vi "_script_import_api_doc.vi"(10 "pattern":string="VI Description(CN) - *", 11 "md path":path) -> ()   [LabVIEW 2017]
uses:
  Communicable State Machine.lvlib
  _csmDoc/csmdoc.lvlib
panel:
  out "States":string
  out "appended array":path[](array[path])
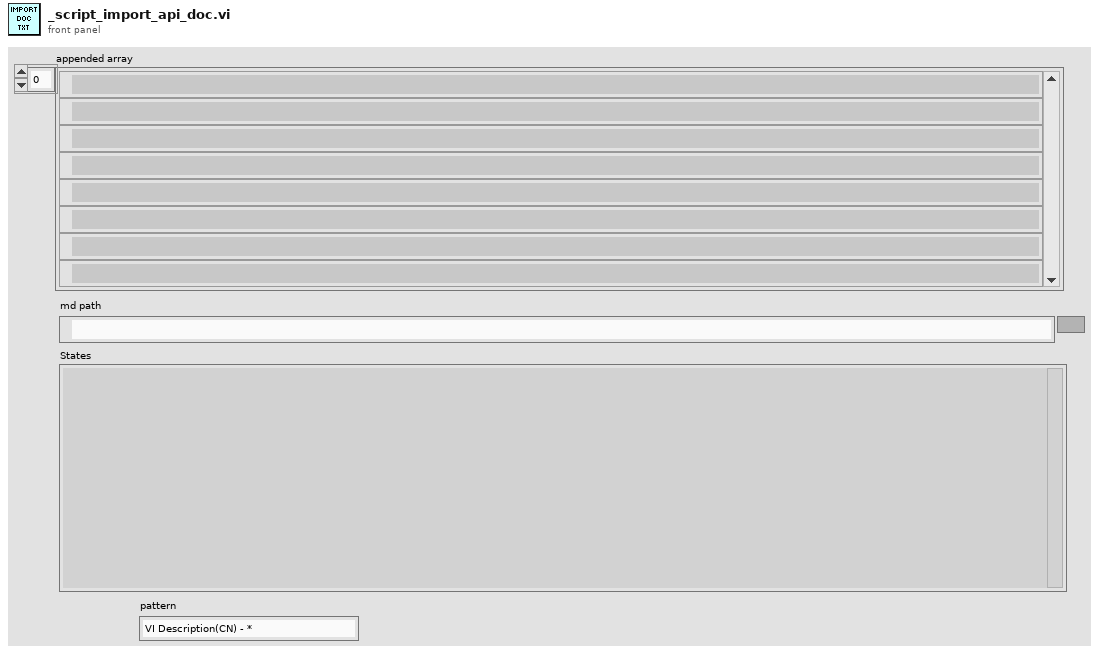
[diagram p1: front panel]
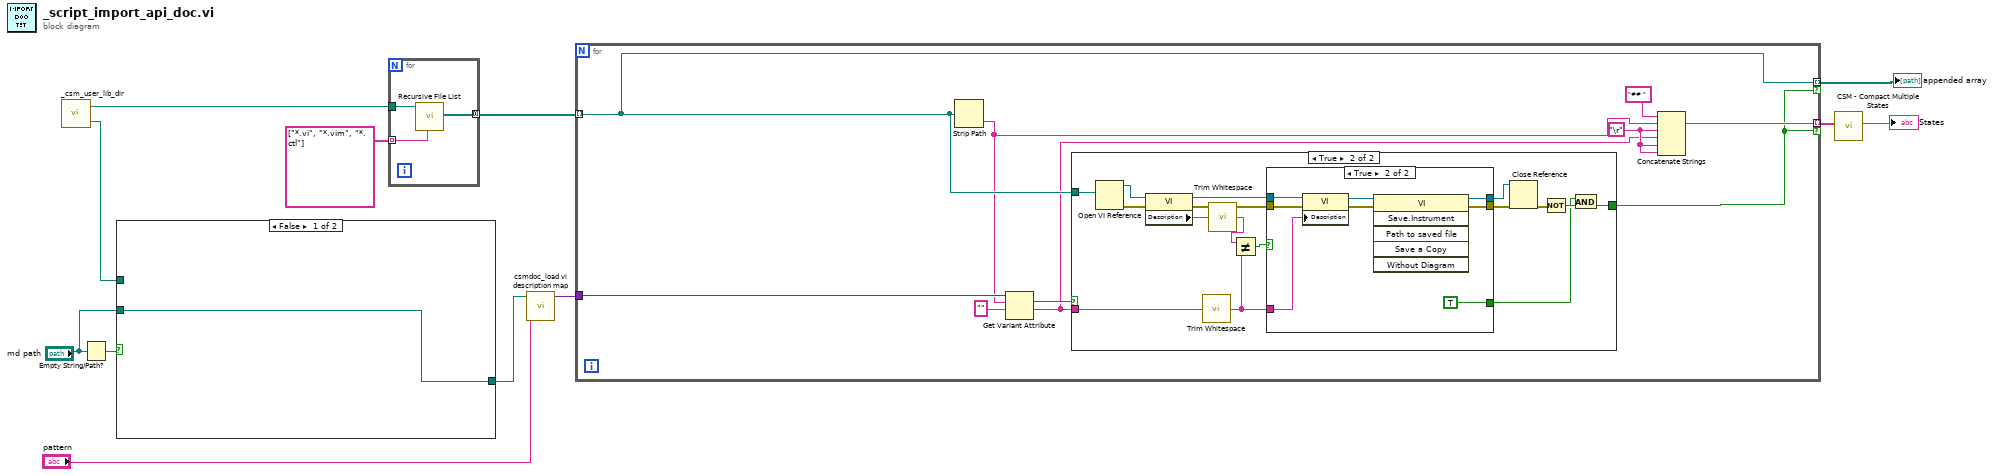
[diagram p0: block diagram]
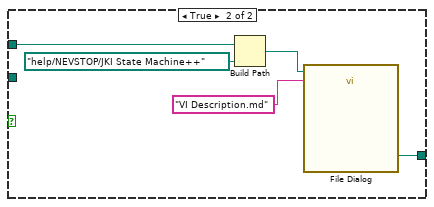
[diagram p2: hidden frame]
diagram:
  n1 = call "_csm_user_lib_dir.vi"() -> ("<LabVIEW>"=w4:path, "csm_user.lib_dir"=w5:path)  [unwired: 2 in]
  n2 = Empty String/Path?(string/path="md path") -> (empty?=w3:bool)
  n3 = case shown="False" w3 {
    tunnel: [w13 w16] -> w8
    tunnel: w4 -> [_ w14]
    tunnel: "md path" -> [w13 _]
    frame False {
    }
    frame True {
      n4 = Build Path(base path=w14, name or relative path=path "help/NEVSTOP/JKI State Machine++" ("Path")) -> (appended path=w17:path)
      n5 = call "File Dialog"("start path"=w17, "default name"="VI Description.md") -> ("selected path"=w16:path)  [unwired: 10 in, 3 out]
    }
  }
  n6 = for {
    tunnel: w5 -> [w21]
    tunnel: string[] ["*.vi", "*.vim", "*.ctl"] -> [w20] mode=indexing
    tunnel: [w19] -> w11 mode=concatenating
    n7 = call <vilib>:"Recursive File List.vi"("pattern"=w20, "Folder Path"=w21) -> ("All Files in Dir"=w19:path[])  [unwired: 5 in, 4 out]
  }
  n8 = call "csmdoc_load vi description map.vi"("pattern"="pattern", "Path"=w8) -> ("variant"=w9:variant)  [unwired: 7 in, 2 out]
  n9 = for {
    tunnel: w11 -> [w29] mode=indexing
    tunnel: [w31] -> w10 mode=indexing if=w30
    tunnel: w9 -> [w28]
    tunnel: [w29] -> w6 mode=indexing if=w30
    w26 = "\r"
    n10 = Strip Path(path=w29) -> (name=w23:string)  [unwired: 1 out]
    n11 = Get Variant Attribute(Variant=w28, name=w23, default value (empty Variant)="" ("string")) -> (found=w24:bool, value=w22:string)  [unwired: 1 in, 2 out]
    n12 = case shown="True" w24 {
      tunnel: w29 -> [_ w47]
      tunnel: w22 -> [_ w46]
      tunnel: [_ w33] -> w30
      frame False {
      }
      frame True {
        n13 = Open VI Reference(vi path=w47) -> (vi reference=w40:refnum<vi>, error out=w41:errorcluster)  [unwired: 5 in]
        n14 = property class="VI"(reference=w40, error in=w41) -> (reference out=w38:refnum<vi>, error out=w39:errorcluster, "Description"=w37:string)
        n15 = call <vilib>:"Trim Whitespace.vi"("string"=w46) -> ("trimmed string"=w35:string)  [unwired: 1 in]
        n16 = call <vilib>:"Trim Whitespace.vi"("string"=w37) -> ("trimmed string"=w36:string)  [unwired: 1 in]
        n17 = Not Equal?(x=w36, y=w35) -> (x != y?=w34:bool)
        n18 = case shown="True" w34 {
          tunnel: [w49 w56] -> w45
          tunnel: [w48 w54] -> w44
          tunnel: w35 -> [_ w53]
          tunnel: w39 -> [w49 w52]
          tunnel: w38 -> [w48 w51]
          tunnel: [_ TRUE] -> w32
          frame False {
          }
          frame True {
            n19 = property class="VI"(reference=w51, error in=w52, "Description"=w53) -> (reference out=w55:refnum<vi>, error out=w57:errorcluster)
            n20 = invoke class="VI" method="Save.Instrument"(reference=w55, error in=w57) -> (reference out=w54:refnum<vi>, error out=w56:errorcluster)  [unwired: 4 in, 4 out]
          }
        }
        n21 = Close Reference(reference=w44, error in (no error)=w45) -> (error out=w43:errorcluster)
        n22 = Not(x=w43) -> (.not. x?=w42:bool)
        n23 = And(x=w32, y=w42) -> (x .and. y?=w33:bool)
      }
    }
    n24 = Concatenate Strings("## " ("string"), w23, w26, w22, w26, w26) -> (w31:string)
  }
  "appended array" <- w6
  n25 = call "CSM - Compact Multiple States.vi"("Multiple States"=w10) -> ("States"=→"States":string)  [unwired: 9 in]
